vi "ExtractArchivedData.vi"() -> ()   [LabVIEW 2014, in "examples.lvlib"]
uses:
  examples.lvlib
  vis/tango_vi.llb/avToDoubleScalarAv.vi
  vis/tango_vi.llb/tango.lvlib
panel:
  out "success":bool
  out "XY Graph":cluster{"Y":dbl[], "Y":dbl[]}[](graph)
  in  "sampling":string="MINUTE"
  in  "to_date":string="2010-02-02 00:00:00"
  in  "from_date":string="2010-02-01 00:00:00"
  in  "archived_attr_name":string="ANS-C03/DG/DCCT/current"
  in  "db_extractor_dev_name":string="archiving/hdbextractor/1"
  out "archived values":dbl[][](array[numeric])
  out "timestamps":dbl[][](array[numeric])
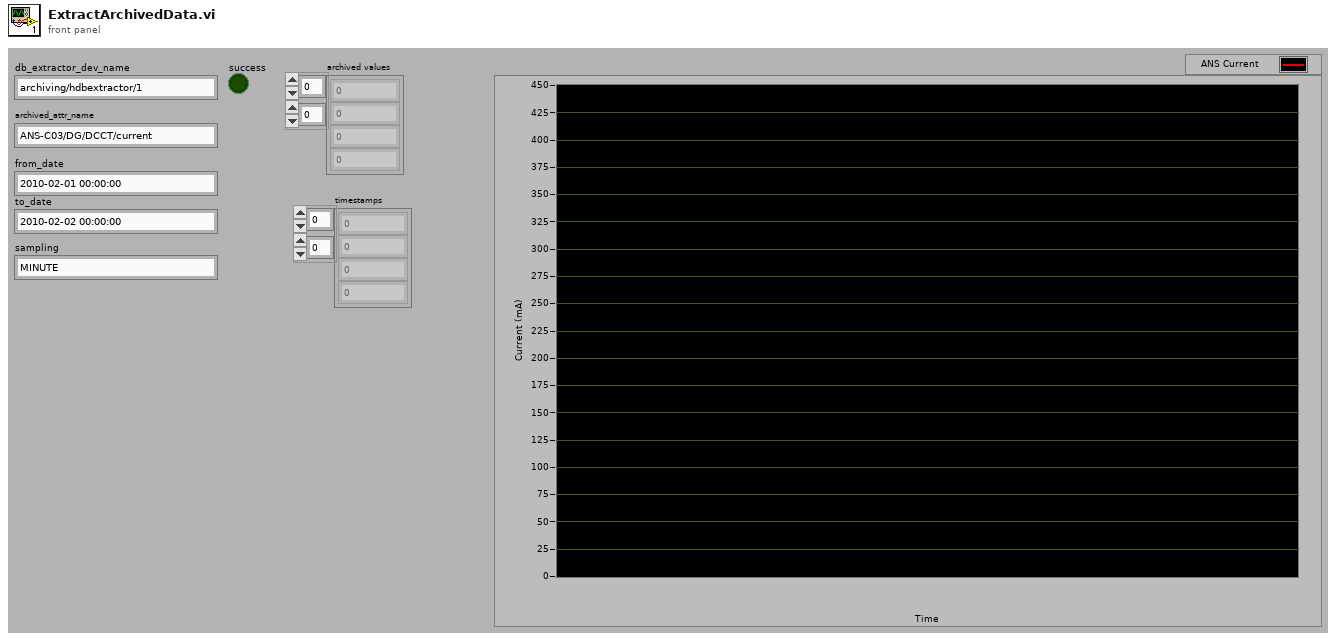
[diagram p1: front panel]
types:
  T1 = typedef "tango.lvlib/_AttributeValue_t.ctl" = cluster{"device name":string, "attribute name":string, "quality value":T2, "quality string":string, "timestamp":dbl, "dim. x":i32, "dim. y":i32, "value":u8[], "error code":i32, "error stack":string[], "data type":T3}
  T2 = typedef "tango.lvlib/_AttributeQuality_t.ctl" = enum16{"VALID", "INVALID", "ALARM", "CHANGING", "UNKNOWN_QUALITY"}
  T3 = typedef "tango.lvlib/_AttributeDataType_t.ctl" = enum16{"STATE_SCA", "STATE_SPE", "STATE_IMG", "STRING_SCA", "STRING_SPE", "STRING_IMG", "BOOL_SCA", "BOOL_SPE", "BOOL_IMG", "UCHAR_SCA", "UCHAR_SPE", "UCHAR_IMG", "SHORT_SCA", "SHORT_SPE", "SHORT_IMG", "USHORT_SCA", "USHORT_SPE", "USHORT_IMG", "LONG_SCA", "LONG_SPE", "LONG_IMG", "ULONG_SCA", "ULONG_SPE", "ULONG_IMG", "LONG64_SCA", "LONG64_SPE", "LONG64_IMG", "ULONG64_SCA", "ULONG64_SPE", "ULONG64_IMG", "FLOAT_SCA", "FLOAT_SPE", "FLOAT_IMG", "DOUBLE_SCA", "DOUBLE_SPE", "DOUBLE_IMG", "ENUM_SCA", "UNKNOWN_DATA_TYPE"}
  T4 = cluster{"device name":string, "attribute name":string, "quality value":i16, "quality string":string, "timestamp":dbl, "dim. x":i32, "dim. y":i32, "value":dbl, "error code":i32, "error stack":string[], "data type":u16}
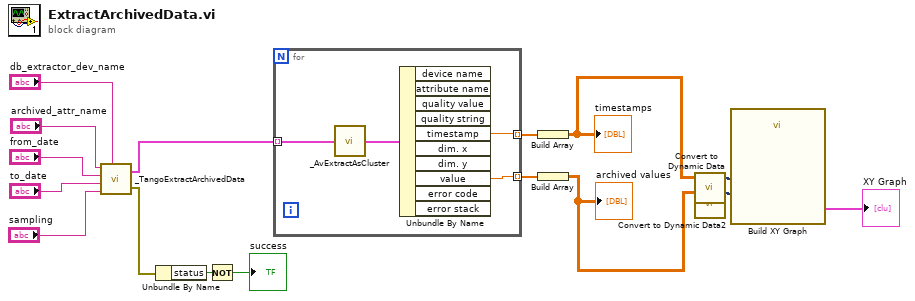
[diagram p0: block diagram]
diagram:
  n1 = call "_TangoExtractArchivedData.vi"("db_extractor_dev_name"="db_extractor_dev_name", "sampling"="sampling", "to_date"="to_date", "from_date"="from_date", "archived_attr_name"="archived_attr_name") -> ("error out"=w3:errorcluster, "attr values"=w11:T1[])  [unwired: 1 in]
  n2 = Unbundle By Name(w3) -> ("status"=w2:bool)
  n3 = Not(x=w2) -> (.not. x?=→"success":bool)
  n4 = for {
    tunnel: w11 -> [w20] mode=indexing
    tunnel: [w18] -> w7 mode=indexing
    tunnel: [w17] -> w5 mode=indexing
    n5 = call-poly "_AvExtractAsCluster.vi"("attribute value"=w20) -> ("av"=w19:T4)
    n6 = Unbundle By Name(w19) -> ("timestamp"=w18:dbl, "value"=w17:dbl)  [unwired: 8 out]
  }
  n7 = Build Array(w7) -> (w6:dbl[][])
  "timestamps" <- w6
  n8 = Build Array(w5) -> (w4:dbl[][])
  "archived values" <- w4
  n9 = call "Convert to Dynamic Data"("2D Array"=w6) -> ("Dynamic Data Type"=w9:dynamicdata)  [unwired: 3 in]
  n10 = call "Convert to Dynamic Data2"("2D Array"=w4) -> ("Dynamic Data Type"=w8:dynamicdata)  [unwired: 3 in]
  n11 = call "Build XY Graph"("Y Input"=w8, "X Input"=w9) -> ("XY Graph"=→"XY Graph":cluster{"Y":dbl[], "Y":dbl[]}[])  [unwired: 8 in, 1 out]
